vi "queue server testing.vi"() -> ()   [LabVIEW 2015]
uses:
  Queue server/Queue server.lvclass
  Queue Client/Queue client.lvclass
  Queue connection/Queue connection.lvclass
  connection/connection maintainer.lvclass
  message/communicator message.lvclass
  communicator manager/communicator manager.lvlib
  communicator/communicator.lvclass
  communicator queue/identifying queue.lvclass
  manager/queue manager.lvclass
panel:
  out "ID 5":string
  out "data 5":variant
  out "queue":refnum<class "identifying queue.lvclass">
  out "data 4":variant
  out "ID 4":string
  out "data 3":variant
  out "ID 3":string
  out "error IO":errorcluster
  out "rawenqerr":errorcluster
  out "valid?":bool
  out "error out 4":errorcluster
  out "error out 3":errorcluster
  out "error out 2":errorcluster
  out "error out":errorcluster
  in  "raw enq":bool
  in  "data 2":string
  in  "ID 2":string
  in  "data":string
  in  "ID":string
  in  "stop":bool
  in  "send":bool
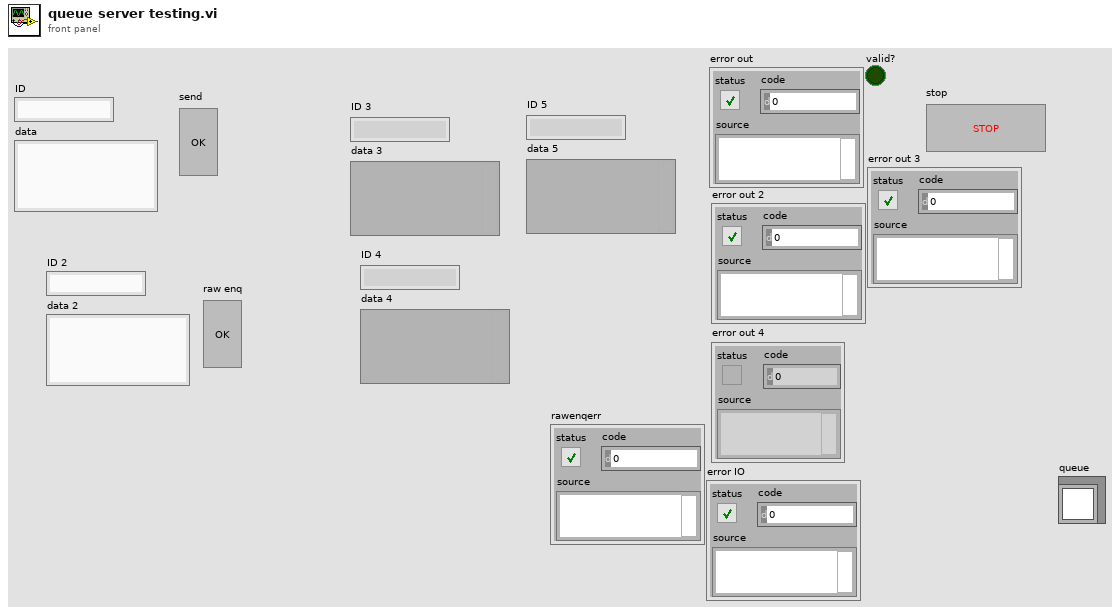
[diagram p1: front panel]
types:
  T1 = typedef "Queue connection.lvclass/queue pair.ctl" = cluster{"to pair":refnum<queue>, "from pair":refnum<queue>}
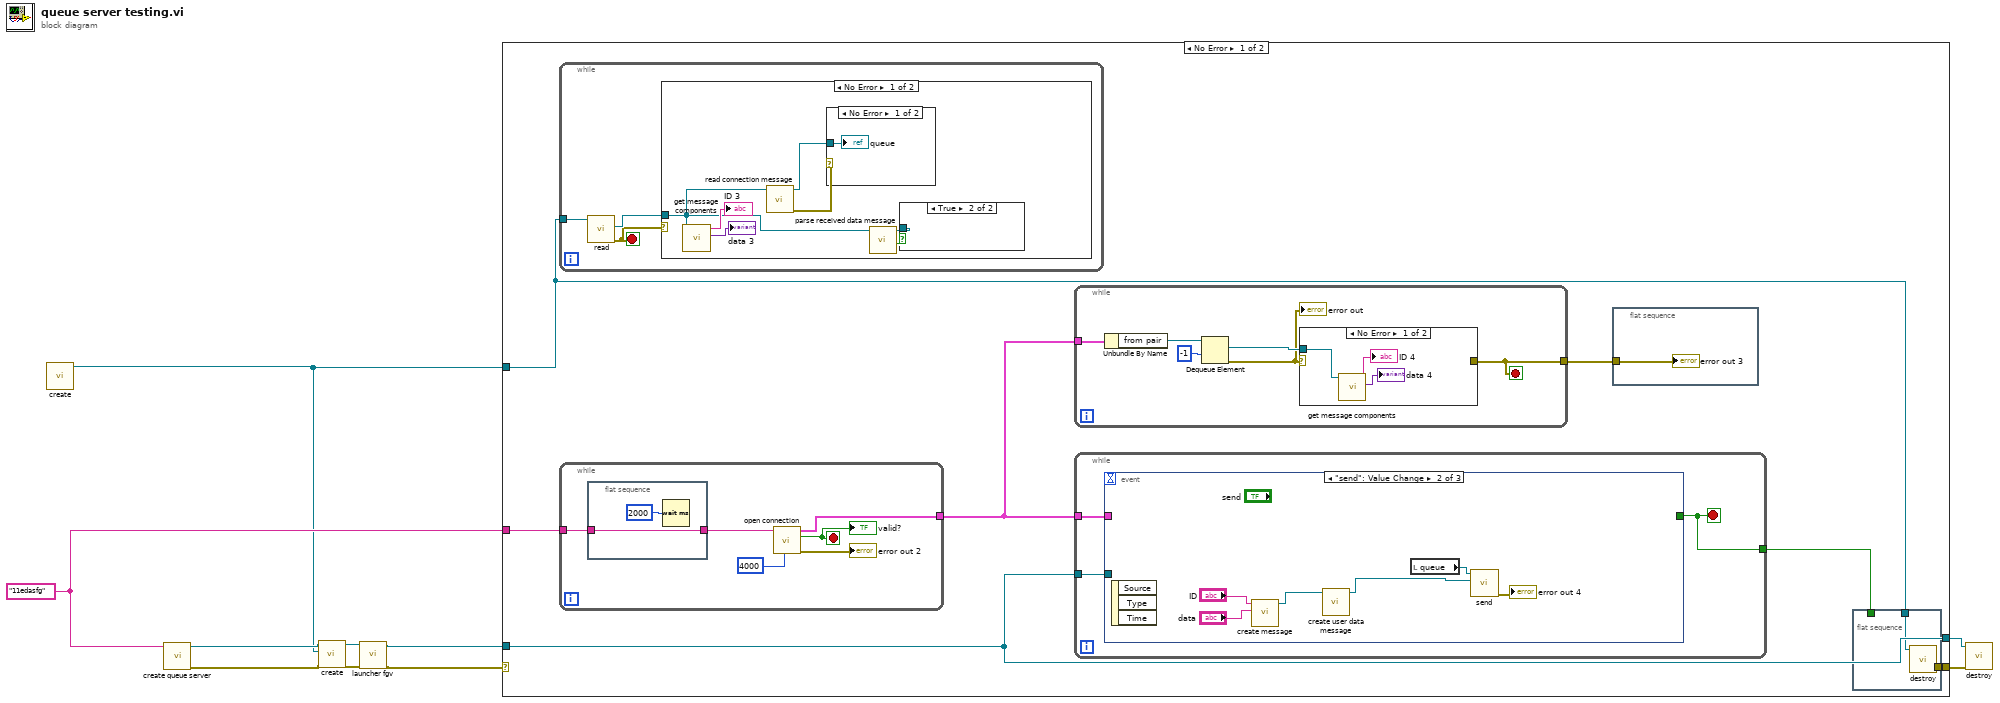
[diagram p0: block diagram]
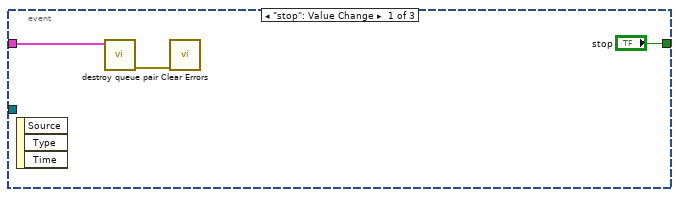
[diagram p3: hidden frame]
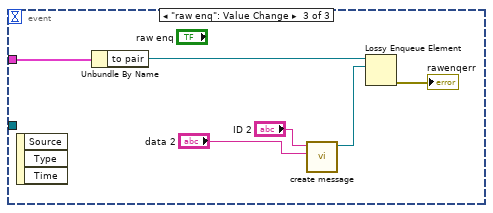
[diagram p4: hidden frame]
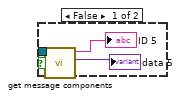
[diagram p5: hidden frame]
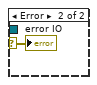
[diagram p7: hidden frame]
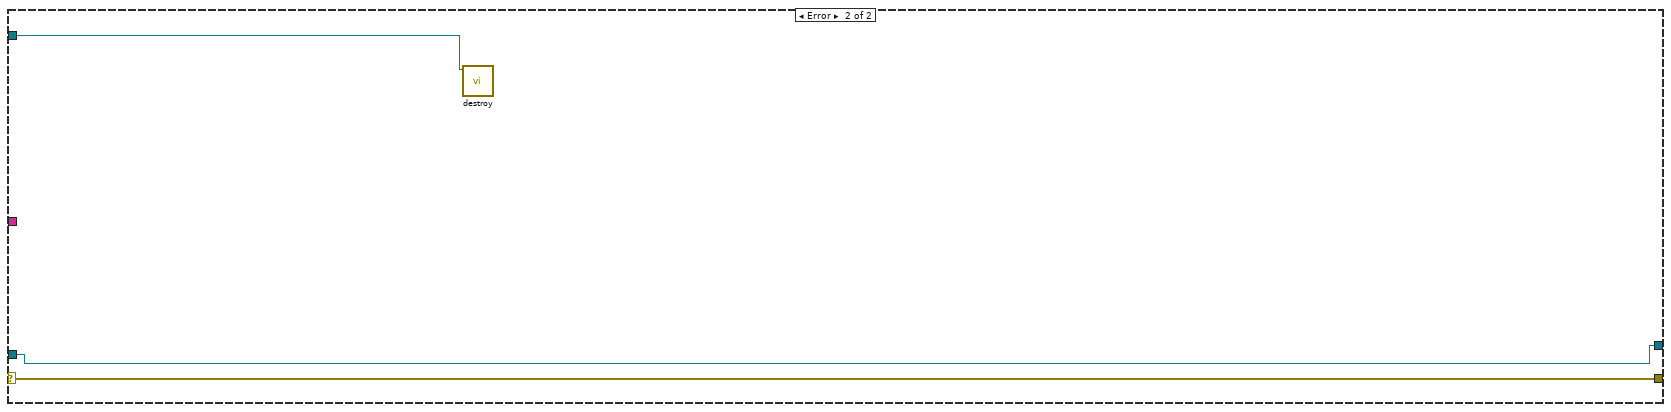
[diagram p8: hidden frame]
diagram:
  w8 = "11edasfg" ("connection string")
  n1 = call "create.vi"() -> ("message connection out"=w1:refnum<class "identifying queue.lvclass">)  [unwired: 10 in, 1 out]
  n2 = call "create queue server.vi"("conn string"=w8) -> ("error out"=w5:errorcluster, "TCP server out"=w2:refnum<class "Queue server.lvclass">)  [unwired: 9 in]
  n3 = call "create.vi"("error in"=w5, "parent"=w1, "uninitialized communicator"=w2) -> ("error out"=w7:errorcluster, "communicator out"=w6:refnum<class "Queue server.lvclass">)  [unwired: 7 in]
  n4 = call "launcher fgv.vi"("error in"=w7, "communicator in"=w6) -> ("error out"=w4:errorcluster, "initialized communicator"=w3:refnum<class "communicator.lvclass">)  [unwired: 8 in]
  n5 = case shown="No Error" w4 {
    selector: w4 -> [_ w75]
    tunnel: [w16 w74] -> w10
    tunnel: [w13 w75] -> w9
    tunnel: w3 -> [w16 w74]
    tunnel: w8 -> [w15 _]
    tunnel: w1 -> [w12 w73]
    frame No Error {
      n6 = while {
        tunnel: w12 -> [w58]
        stop <- w59 stop-if-true
        n7 = call "read.vi"("identifying queue in"=w58) -> ("error out"=w59:errorcluster, "message"=w60:refnum<class "communicator message.lvclass">)  [unwired: 8 in, 1 out]
        n8 = case shown="No Error" w59 {
          selector: w59 -> [_ w72]
          tunnel: w60 -> [w63 _]
          frame No Error {
            n9 = call "get message components.vi"("message"=w63) -> ("data"=→"data 3":variant, "ID"=→"ID 3":string)  [unwired: 9 in]
            n10 = call "read connection message.vi"("communicator message in"=w63) -> ("error out"=w67:errorcluster, "queue"=w66:refnum<class "identifying queue.lvclass">)  [unwired: 9 in]
            n11 = case shown="No Error" w67 {
              tunnel: w66 -> [w71 _]
              frame No Error {
                "queue" <- w71
              }
              frame Error {
              }
            }
            n12 = call "parse received data message.vi"("message"=w63) -> ("invalid?"=w61:bool, "data"=w62:refnum<class "communicator message.lvclass">)  [unwired: 9 in]
            n13 = case shown="True" w61 {
              tunnel: w62 -> [w70 _]
              frame False {
                n14 = call "get message components.vi"("message"=w70) -> ("data"=→"data 5":variant, "ID"=→"ID 5":string)  [unwired: 9 in]
              }
              frame True {
              }
            }
          }
          frame Error {
            "error IO" <- w72
          }
        }
      }
      n15 = while {
        tunnel: w15 -> [w26]
        tunnel: [w22] -> w14
        stop <- w23 stop-if-true
        n16 = flat-sequence {
          tunnel: [w27] -> w25
          tunnel: w26 -> [w27]
          frame #0 {
            n17 = Wait (ms)(milliseconds to wait=u32 2000) -> ()  [unwired: 1 out]
          }
        }
        n18 = call "open connection.vi"("timeout ms (10000)"=4000, "address"=w25) -> ("error out"=→"error out 2":errorcluster, "valid?"=w23:bool, "output cluster"=w22:T1)  [unwired: 7 in]
        "valid?" <- w23
      }
      n19 = while {
        tunnel: w14 -> [w33]
        tunnel: [w32] -> w17
        stop <- w32 stop-if-true
        n20 = Unbundle By Name(w33) -> ("from pair"=w31:refnum<queue>)
        n21 = Dequeue Element(queue=w31, timeout in ms (-1)=-1 ("timeout ms (25000)")) -> (element=w35:refnum<class "communicator message.lvclass">, error out=w30:errorcluster)  [unwired: 1 in, 2 out]
        "error out" <- w30
        n22 = case shown="No Error" w30 {
          selector: w30 -> [_ w39]
          tunnel: [_ w39] -> w32
          tunnel: w35 -> [w38 _]
          frame No Error {
            n23 = call "get message components.vi"("message"=w38) -> ("data"=→"data 4":variant, "ID"=→"ID 4":string)  [unwired: 9 in]
          }
          frame Error {
          }
        }
      }
      n24 = while {
        tunnel: w16 -> [w42]
        tunnel: w14 -> [w41]
        tunnel: [w40] -> w11
        stop <- w40 stop-if-true
        n25 = event shown="[1] \"send\": Value Change" {
          selector: _ -> [_ _ _]
          dyn-events: _ -> [_ _ _]
          timeout: _ -> [_ _ _]
          tunnel: ["stop" _ _] -> w40
          tunnel: w42 -> [_ _ _]
          tunnel: w41 -> [w44 _ w57]
          event "stop": Value Change {
            n26 = event-data() -> ()  [unwired: 1 in, 3 out]
            n27 = call "destroy queue pair.vi"("queue connection"=w44) -> ("error out"=w43:errorcluster)  [unwired: 10 in]
            n28 = call <vilib>:"Clear Errors.vi"("error in (no error)"=w43) -> ()  [unwired: 5 in, 2 out]
          }
          event "send": Value Change {
            n29 = event-data() -> ()  [unwired: 1 in, 3 out]
            n30 = call "create message.vi"("data"="data", "ID"="ID") -> ("message"=w47:refnum<class "communicator message.lvclass">)  [unwired: 9 in]
            n31 = call "create user data message.vi"("data"=w47) -> ("message"=w46:refnum<class "communicator message.lvclass">)  [unwired: 10 in]
            n32 = local read "queue"() -> (w51:refnum<class "identifying queue.lvclass">)
            n33 = call "send.vi"("message"=w46, "message connection in"=w51) -> ("error out"=→"error out 4":errorcluster)  [unwired: 8 in, 1 out]
          }
          event "raw enq": Value Change {
            n34 = event-data() -> ()  [unwired: 1 in, 3 out]
            n35 = Unbundle By Name(w57) -> ("to pair"=w56:refnum<queue>)
            n36 = call "create message.vi"("data"="data 2", "ID"="ID 2") -> ("message"=w54:refnum<class "communicator message.lvclass">)  [unwired: 9 in]
            n37 = Lossy Enqueue Element(queue=w56, element=w54) -> (error out=→"rawenqerr":errorcluster)  [unwired: 1 in, 3 out]
          }
        }
      }
      n38 = flat-sequence {
        tunnel: w17 -> [w29]
        frame #0 {
          "error out 3" <- w29
        }
      }
      n39 = flat-sequence {
        tunnel: [w20] -> w13
        tunnel: w12 -> [w19]
        tunnel: [w18] -> _
        tunnel: w11 -> [w18]
        frame #0 {
          n40 = call "destroy.vi"("message connection in"=w19) -> ("error out"=w20:errorcluster)  [unwired: 10 in]
        }
      }
    }
    frame Error {
      n41 = call "destroy.vi"("message connection in"=w73) -> ()  [unwired: 10 in, 1 out]
    }
  }
  n42 = call-dynamic "destroy.vi"("error in"=w9, "communicator in"=w10) -> ()  [unwired: 9 in, 1 out]
